vi "FPGA_Main_Test.vi"() -> ()   [LabVIEW 2019]
uses:
  <vilib>/FPGAPlugInAG/myRIO-1900/niLvFpga_Open_myRIO-1900.vi
  <vilib>/rvi/interface/common/dynamic/niFpgaDynamicAddResources.vi
  <vilib>/Utility/error.llb/Error Cluster From Error Code.vi
  <vilib>/rvi/errors/niLvFpgaAdjustHostInterfaceError.vi
  <vilib>/rvi/interface/nirviOpenFPGA/nirviOpenFPGA.xnode
  FPGA Bitfiles/ascenceur_FPGATarget_FPGAMain_7v9Jr2n8zuw.lvbitx
  FPGA_Main.vi
  <vilib>/rvi/interface/nirviReadWriteControl/nirviReadWriteControl.xnode
  NiFpgaLv.dll
  <vilib>/rvi/interface/Simulation/niFpgaSimulationCallBeginRW.vi
panel:
  in  "Porte  3":enum16{"Monter", "Descendre", "Arreter"}(ring)
  in  "Porte  2":enum16{"Monter", "Descendre", "Arreter"}(ring)
  in  "Porte  1":enum16{"Monter", "Descendre", "Arreter"}(ring)
  in  "Porte RDC":enum16{"Monter", "Descendre", "Arreter"}(ring)
  in  "CMD_Moteur_Cabine":enum16{"Monter", "Descendre", "Arreter"}(ring)
  out "Portes_Ouvertes":bool[](array[boolean])
  out "Portes_Fermees":bool[](array[boolean])
  out "Presence_Cabine":bool[](array[boolean])
  in  "Bouton Stop":bool
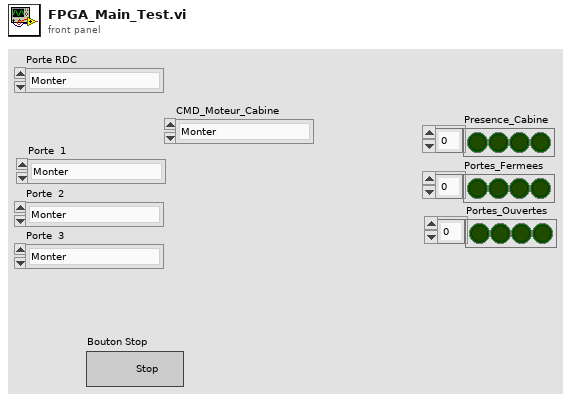
[diagram p1: front panel]
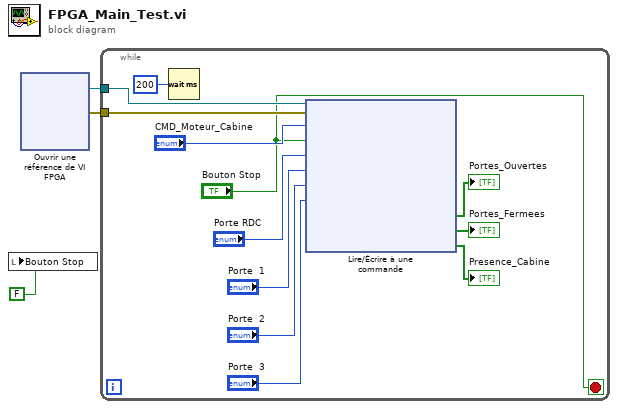
[diagram p0: block diagram]
diagram:
  n1 = local write "Bouton Stop"(FALSE ("Bouton Stop")) -> ()
  n2 = xnode "Ouvrir une référence de VI FPGA"() -> ("Référence de VI FPGA en sortie"=w3:refnum<k20>, "sortie d'erreur"=w2:errorcluster)  [unwired: 2 in]
  n3 = while {
    tunnel: w3 -> [w15]
    tunnel: w2 -> [w14]
    stop <- "Bouton Stop" stop-if-true
    n4 = Wait (ms)(milliseconds to wait=u32 200 ("attente (ms)")) -> ()  [unwired: 1 out]
    n5 = xnode "Lire/Écrire à une commande"("Référence de VI FPGA en entrée"=w15, "entrée d'erreur"=w14, "CMD_Moteur_Cabine"="CMD_Moteur_Cabine", "STOP"="Bouton Stop", "CMD_Moteur_Porte_RDC"="Porte RDC", "CMD_Moteur_Porte_1"="Porte  1", "CMD_Moteur_Porte_2"="Porte  2", "CMD_Moteur_Porte_3"="Porte  3") -> ("Portes_Ouvertes"=→"Portes_Ouvertes":bool[], "Portes_Fermees"=→"Portes_Fermees":bool[], "Presence_Cabine"=→"Presence_Cabine":bool[])  [unwired: 2 out]
  }
